vi "convert to extended UTC.vi"(1 "Real UTC":dbl format="%<%H:%M:%S>t") -> (0 "extended UTC":dbl format="%<%H:%M:%S>t")   [LabVIEW 2011]
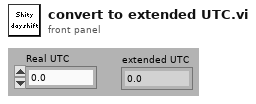
[diagram p1: front panel]
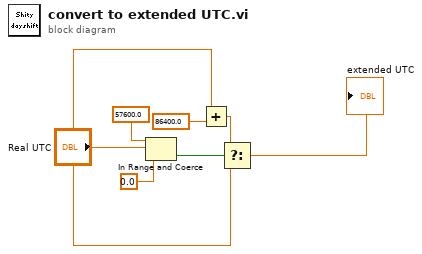
[diagram p0: block diagram]
diagram:
  n1 = In Range and Coerce(upper limit=57600.0 ("x"), x="Real UTC", lower limit=0.0 ("x")) -> (In Range?=w5:bool)  [unwired: 1 out]
  n2 = Add(x="Real UTC", y=86400.0) -> (x+y=w4:dbl)
  n3 = Select(t=w4, s=w5, f="Real UTC") -> (s? t:f=→"extended UTC":dbl)
